vi "main.vi"() -> ()   [LabVIEW 2018]
uses:
  <vilib>/Analysis/NI_AALBase.lvlib
  <vilib>/Analysis/baseanly.llb/Real Inverse Matrix.vi
  <vilib>/robotics/Kinematics/Quaternion.ctl
  <vilib>/robotics/Kinematics/NI_Kinematics.lvlib
  <vilib>/imathl/engines/lvmath/Functions/Error Handling/Create Error.vi
  <vilib>/imath/engines/lvmath2/RunTimeEngine/IndexRead/NIMS V(S).vi
  <vilib>/imath/engines/lvmath2/RunTimeEngine/NodeEndStatement/NIMS_NodeEndStatement_Output.vi
  <vilib>/imath/engines/lvmath2/RunTimeEngine/ErrorHandling/NIMS_Finalize Error.vi
  <vilib>/imath/engines/lvmath2/RunTimeEngine/IndexRead/NIMS V(R2).vi
  <vilib>/imath/engines/lvmath2/RunTimeEngine/BuiltInFunctions/mean/NIMS_RS=mean(RV,I32).vi
  <vilib>/imath/engines/lvmath2/RunTimeEngine/IndexRead/NIMS M($,S).vi
  <vilib>/imath/engines/lvmath2/RunTimeEngine/RowToken/NIMS_RowToken_SorRV_CV.vi
panel:
  out "avg_er3":dbl
  out "avg_er2":dbl
  out "avg_er1":dbl
  out "eR (Yaw)":cluster{"E1_now":dbl[], "t_now":dbl[]}(graph)
  out "eR (Pitch)":cluster{"E1_now":dbl[], "t_now":dbl[]}(graph)
  out "eR (Roll)":cluster{"E1_now":dbl[], "t_now":dbl[]}(graph)
  out "Yaw":cluster{"E1_now":dbl[], "t_now":dbl[]}(graph)
  out "Pitch":cluster{"E1_now":dbl[], "t_now":dbl[]}(graph)
  out "Roll":cluster{"E1_now":dbl[], "t_now":dbl[]}(graph)
  in  "Simulation Time (sec)":dbl
  in  "Systems Configuration":T1
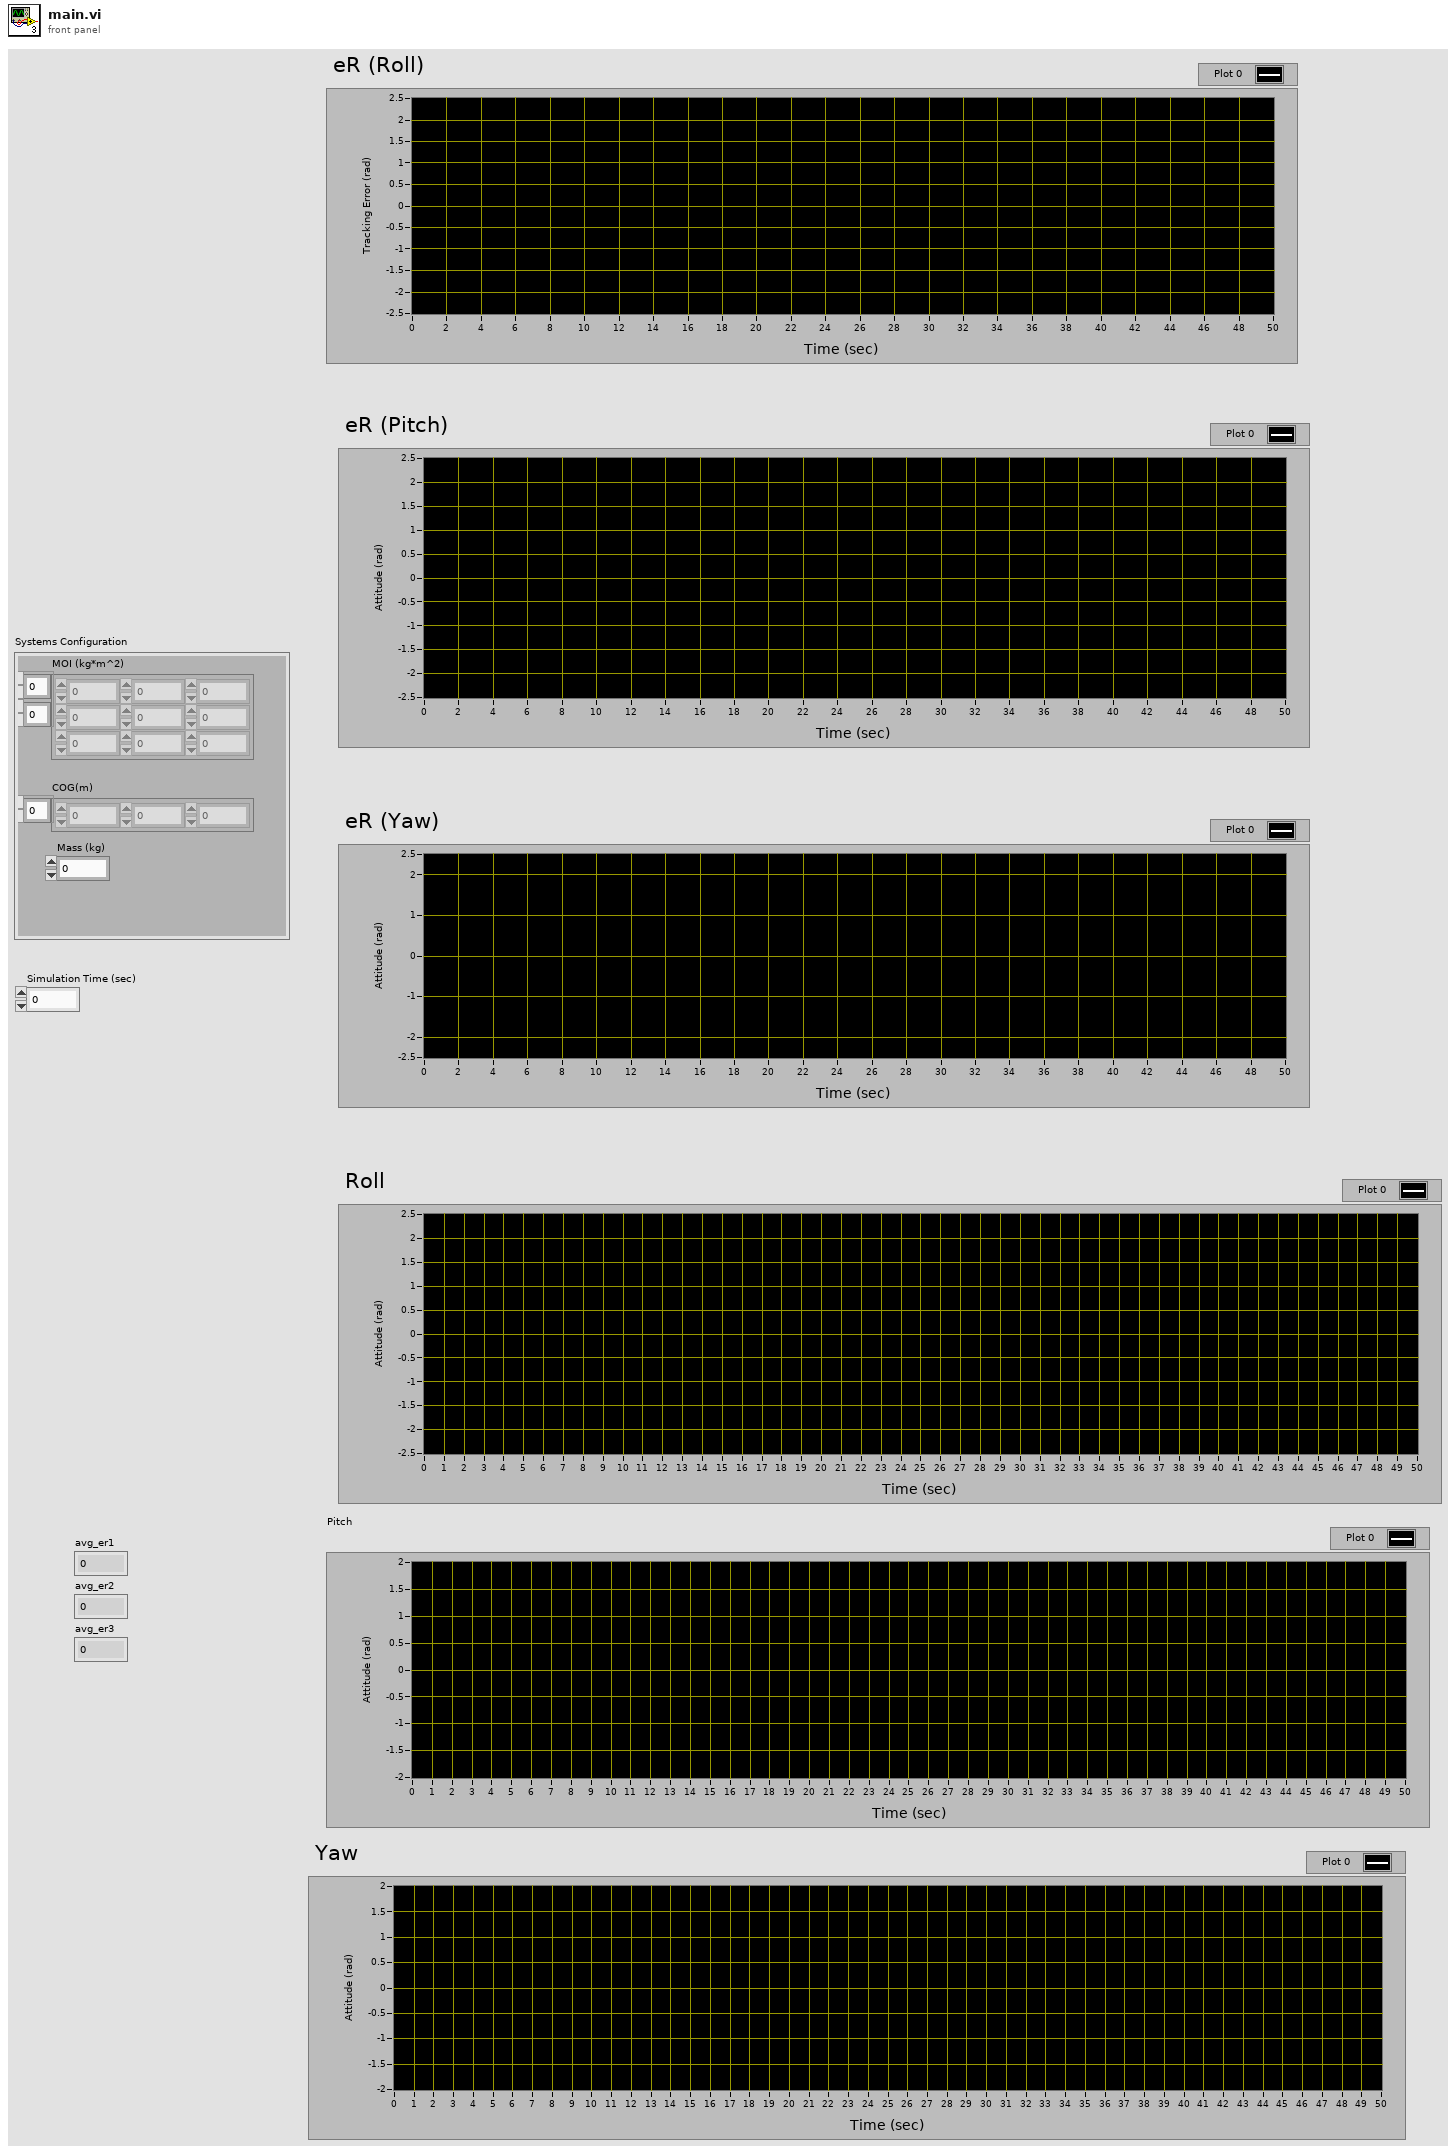
[diagram p1: front panel]
types:
  T1 = cluster{"MOI (kg*m^2)":dbl[][], "Mass (kg)":dbl, "COG(m)":dbl[]}
  T2 = typedef "NI_Matrix.lvlib/RealMatrix.ctl" = dbl[][]
  T3 = cluster{"MOI (kg*m^2)":dbl[][], "Inverse Matrix":T2, "Mass (kg)":dbl, "COG(m)":dbl[]}
  T4 = typedef "NI_Kinematics.lvlib/Quaternion.ctl" = dbl[]
  T5 = cluster{"E1_now":dbl[], "E2_now":dbl[], "E3_now":dbl[], "t_now":dbl[]}
  T6 = cluster{"Er1":dbl[], "Er2":dbl[], "Er3":dbl[], "t_now":dbl[]}
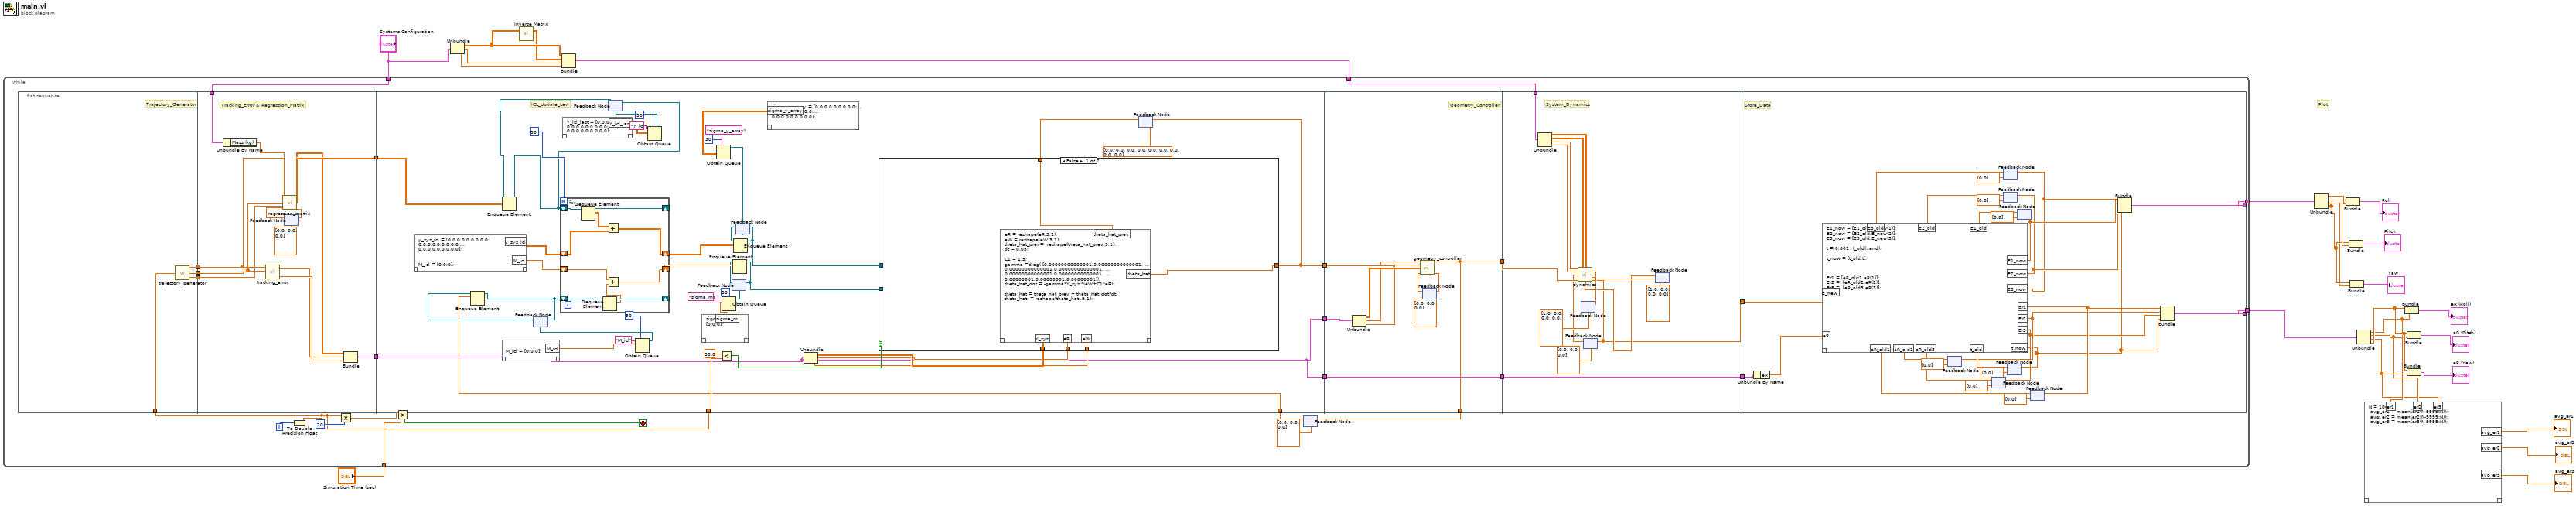
[diagram p0: block diagram]
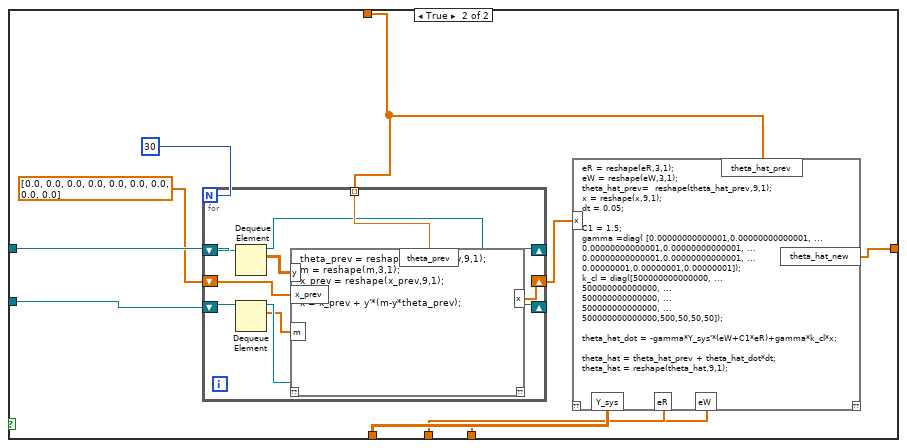
[diagram p2: hidden frame]
diagram:
  # "Plot"
  n1 = Unbundle("Systems Configuration") -> ("MOI (kg*m^2)"=w24:dbl[][], "Mass (kg)"=w22:dbl, "COG(m)"=w21:dbl[])
  n2 = call-poly <vilib>:"Inverse Matrix.vi"("Input Matrix"=w24) -> ("Inverse Matrix"=w23:T2)  [unwired: 1 in, 1 out]
  n3 = Bundle("MOI (kg*m^2)"=w24, "Inverse Matrix"=w23, "Mass (kg)"=w22, "COG(m)"=w21) -> (w20:T3)  [unwired: 1 in]
  n4 = while {
    tunnel: "Simulation Time (sec)" -> [w49]
    tunnel: "Systems Configuration" -> [w44]
    tunnel: w20 -> [w36]
    tunnel: [w31] -> w12
    tunnel: [w30] -> w1
    i -> [w47]
    stop <- w48 stop-if-true
    n5 = flat-sequence {
      tunnel: w41 -> [w55]
      tunnel: [w54] -> w46
      tunnel: [w53] -> w45
      tunnel: [w52] -> w43
      tunnel: w46 -> [w63]
      tunnel: w45 -> [w62]
      tunnel: w44 -> [w68]
      tunnel: w43 -> [w61]
      tunnel: [w60] -> w42
      tunnel: [w56] -> w40
      tunnel: w42 -> [w109]
      tunnel: w41 -> [w105]
      tunnel: w40 -> [w70]
      tunnel: [w70] -> w39
      tunnel: [w71] -> w38
      tunnel: [w70] -> w34
      tunnel: w28 -> [w69]
      tunnel: w39 -> [w153]
      tunnel: w38 -> [w148]
      tunnel: [w144] -> w37
      tunnel: w34 -> [w145]
      tunnel: [w145] -> w33
      tunnel: [w144] -> w29
      tunnel: w37 -> [w168]
      tunnel: w36 -> [w167]
      tunnel: [w155] -> w35
      tunnel: w33 -> [w154]
      tunnel: [w154] -> w32
      tunnel: w35 -> [w192]
      tunnel: w32 -> [w194]
      tunnel: [w170] -> w31
      tunnel: [w169] -> w30
      frame #0 {
        # "Trajectory_Generator"
        n6 = call "trajectory_generator.vi"("T"=w55) -> ("Ed"=w54:dbl[], "desired_angular_velocity"=w53:dbl[], "desired_angular_acceleration"=w52:dbl[])
      }
      frame #1 {
        # "Tracking_Error & Regression_Matrix"
        n7 = Unbundle By Name(w68) -> ("Mass (kg)"=w67:dbl)
        n8 = call "tracking_error.vi"("Ed(\"ZYX\")"=w63, "Wd"=w62) -> ("eR"=w58:dbl[], "eW"=w59:dbl[])  [unwired: 3 in]
        n9 = feedback #1(dbl[] [0.0, 0.0, 0.0] ("W_Prev")) -> (w65:dbl[])
        n10 = call "regression_matrix.vi"("m"=w67, "Ed"=w63, "Wd"=w62, "Wd_dot"=w61, "W_prev"=w65) -> ("Y_sys"=w57:dbl[][], "Y_icl_sys"=w60:dbl[][], "W_Prev"=w66:dbl[])  [unwired: 20 in]
        n11 = feedback-in #1(w66) -> ()
        n12 = Bundle("Y_sys"=w57, "eR"=w58, "eW"=w59) -> (w56:cluster{"Y_sys":dbl[][], "eR":dbl[], "eW":dbl[]})  [unwired: 1 in]
      }
      frame #2 {
        # "ICL_Update_Law"
        n13 = mathscript code="y_sys_icl = [0,0,0,0,0,0,0,0,0;...\n0,0,0,0,0,0,0,0,0;...\n0,0,0,0,0,0,0,0,0];\n\n\nM_icl = [0;0;0];"() -> ("y_sys_icl"=w107:dbl[][], "M_icl"=w106:dbl[])  [unwired: 1 in, 1 out]
        n14 = mathscript code="M_icl = [0;0;0];"() -> ("M_icl"=w95:dbl[])  [unwired: 1 in, 1 out]
        n15 = mathscript code="Y_icl_last = [0,0,0,0,0,0,0,0,0;...\n0,0,0,0,0,0,0,0,0;...\n0,0,0,0,0,0,0,0,0];"() -> ("Y_icl_last"=w100:dbl[][])  [unwired: 1 in, 1 out]
        n16 = Obtain Queue(max queue size (-1, unlimited)=30, name (unnamed)="M_icl", element data type=w95) -> (queue out=w94:refnum<queue>)  [unwired: 2 in, 2 out]
        n17 = feedback #2(w94) -> (w89:refnum<queue>)
        n18 = Enqueue Element(queue=w89, element=w69) -> (queue out=w90:refnum<queue>)  [unwired: 2 in, 2 out]
        n19 = feedback-in #2(w90) -> ()
        n20 = Obtain Queue(max queue size (-1, unlimited)=30, name (unnamed)="Y_icl", element data type=w100) -> (queue out=w99:refnum<queue>)  [unwired: 2 in, 2 out]
        n21 = feedback #3(w99) -> (w96:refnum<queue>)
        n22 = Enqueue Element(queue=w96, element=w109) -> (queue out=w91:refnum<queue>)  [unwired: 2 in, 2 out]
        n23 = for {
          N: 30 -> [_]
          shift-right: [w139] -> _
          shift-left: w91 -> [w143]
          shift-right: [w140] -> w102
          shift-left: w107 -> [w141]
          shift-right: [w137] -> w101
          shift-left: w106 -> [w138]
          shift-right: [w136] -> _
          shift-left: w90 -> [w135]
          n24 = Dequeue Element(queue=w143) -> (queue out=w139:refnum<queue>, element=w142:dbl[][])  [unwired: 2 in, 2 out]
          n25 = Dequeue Element(queue=w135) -> (queue out=w136:refnum<queue>, element=w134:dbl[])  [unwired: 2 in, 2 out]
          n26 = Add(x=w142, y=w141) -> (x+y=w140:dbl[][])
          n27 = Add(x=w138, y=w134) -> (x+y=w137:dbl[])
        }
        n28 = feedback-in #3(w91) -> ()
        n29 = mathscript code="sigma_m = [0;0;0];"() -> ("sigma_m"=w79:dbl[])  [unwired: 1 in, 1 out]
        n30 = Less?(x=30.0, y=w105) -> (x < y?=w103:bool)
        n31 = Obtain Queue(max queue size (-1, unlimited)=30, name (unnamed)="sigma_m", element data type=w79) -> (queue out=w80:refnum<queue>)  [unwired: 2 in, 2 out]
        n32 = feedback #4(w80) -> (w83:refnum<queue>)
        n33 = Enqueue Element(queue=w83, element=w101) -> (queue out=w72:refnum<queue>)  [unwired: 2 in, 2 out]
        n34 = feedback-in #4(w72) -> ()
        n35 = mathscript code="sigma_y_array = [0,0,0,0,0,0,0,0,0;...\n0,0,0,0,0,0,0,0,0;...\n0,0,0,0,0,0,0,0,0];"() -> ("sigma_y_array"=w88:dbl[][])  [unwired: 1 in, 1 out]
        n36 = Obtain Queue(max queue size (-1, unlimited)=30, name (unnamed)="sigma_y_array", element data type=w88) -> (queue out=w85:refnum<queue>)  [unwired: 2 in, 2 out]
        n37 = feedback #5(w85) -> (w84:refnum<queue>)
        n38 = Enqueue Element(queue=w84, element=w102) -> (queue out=w73:refnum<queue>)  [unwired: 2 in, 2 out]
        n39 = feedback-in #5(w73) -> ()
        n40 = Unbundle(w70) -> ("Y_sys"=w78:dbl[][], "eR"=w77:dbl[], "eW"=w76:dbl[])
        n41 = feedback #6(dbl[] [0.0, 0.0, 0.0, 0.0, 0.0, 0.0, 0.0, 0.0, 0.0] ("theta_hat")) -> (w74:dbl[])
        n42 = case shown="False" w103 {
          tunnel: w78 -> [w114 w124]
          tunnel: w77 -> [w113 w123]
          tunnel: w76 -> [w112 w122]
          tunnel: w74 -> [w111 w118]
          tunnel: w73 -> [_ w121]
          tunnel: w72 -> [_ w120]
          tunnel: [w110 w115] -> w71
          frame False {
            n43 = mathscript code="eR = reshape(eR,3,1);\neW = reshape(eW,3,1);\ntheta_hat_prev=  reshape(theta_hat_prev,9,1);\ndt = 0.05;\n\nC1 = 1.5;\ngamma =diag( [0.00000000000001,0.00000000000001, ...\n0.00000000000001,0.00000000000001, ...\n0.00000000000001,0.00000000000001, ...\n0.00000001,0.00000001,0.00000001]);\ntheta_hat_dot = -gamma*Y_sys'*(eW+C1*eR);\n\ntheta_hat = theta_hat_prev + theta_hat_dot*dt;\ntheta_hat  = reshape(theta_hat ,9,1);"("Y_sys"=w114, "eR"=w113, "eW"=w112, "theta_hat_prev"=w111) -> ("theta_hat"=w110:dbl[])  [unwired: 1 in, 1 out]
          }
          frame True {
            n44 = for {
              N: 30 -> [_]
              shift-right: [w130] -> _
              shift-left: w121 -> [w133]
              shift-right: [w129] -> _
              shift-left: w120 -> [w132]
              tunnel: w118 -> [w131] mode=indexing
              shift-right: [w125] -> w116
              shift-left: dbl[] [0.0, 0.0, 0.0, 0.0, 0.0, 0.0, 0.0, 0.0, 0.0] -> [w126]
              n45 = Dequeue Element(queue=w133) -> (queue out=w130:refnum<queue>, element=w128:dbl[][])  [unwired: 2 in, 2 out]
              n46 = Dequeue Element(queue=w132) -> (queue out=w129:refnum<queue>, element=w127:dbl[])  [unwired: 2 in, 2 out]
              n47 = mathscript code="theta_prev = reshape(theta_prev,9,1);\nm = reshape(m,3,1);\nx_prev = reshape(x_prev,9,1);\n\nx = x_prev + y'*(m-y*theta_prev);"("theta_prev"=w131, "y"=w128, "m"=w127, "x_prev"=w126) -> ("x"=w125:dbl[])  [unwired: 1 in, 1 out]
            }
            n48 = mathscript code="eR = reshape(eR,3,1);\neW = reshape(eW,3,1);\ntheta_hat_prev=  reshape(theta_hat_prev,9,1);\nx = reshape(x,9,1);\ndt = 0.05;\n\nC1 = 1.5;\ngamma =diag( [0.00000000000001,0.00000000000001, ...\n0.00000000000001,0.00000000000001, ...\n0.00000000000001,0.00000000000001, ...\n0.00000001,0.00000001,0.00000001]);\nk_cl = diag([500000000000000, ...\n500000000000000, ...\n500000000000000, ...\n500000000000000, ...\n500000000000000,500,50,50,50]);\n\ntheta_hat_dot = -gamma*Y_sys'*(eW+C1*eR)+gamma*k_cl*x;\n\ntheta_hat = theta_hat_prev + theta_hat_dot*dt;\ntheta_hat = reshape(theta_hat,9,1);"("Y_sys"=w124, "eR"=w123, "eW"=w122, "theta_hat_prev"=w118, "x"=w116) -> ("theta_hat_new"=w115:dbl[])  [unwired: 1 in, 1 out]
          }
        }
        n49 = feedback-in #6(w71) -> ()
      }
      frame #3 {
        # "Geometry_Controller"
        n50 = Unbundle(w153) -> ("Y_sys"=w152:dbl[][], "eR"=w146:dbl[], "eW"=w151:dbl[])
        n51 = feedback #7(dbl[] [0.0, 0.0, 0.0] ("Omega_now")) -> (w149:dbl[])
        n52 = call "geometry_controller.vi"("eR"=w146, "eW"=w151, "Y_sys"=w152, "theta_hat"=w148, "Omga_prev"=w149) -> ("M"=w144:dbl[], "Omega_now"=w150:dbl[])  [unwired: 9 in]
        n53 = feedback-in #7(w150) -> ()
      }
      frame #4 {
        # "System_Dynamics"
        n54 = Unbundle(w167) -> ("MOI (kg*m^2)"=w166:dbl[][], "Inverse Matrix"=w165:T2, "Mass (kg)"=w164:dbl, "COG(m)"=w163:dbl[])
        n55 = feedback #8(dbl[] [1.0, 0.0, 0.0, 0.0] ("W")) -> ()  [unwired: 1 in]
        n56 = feedback #9(dbl[] [0.0, 0.0, 0.0] ("E")) -> (w157:dbl[])
        n57 = feedback #10(T4 [1.0, 0.0, 0.0, 0.0] ("unit quaternion")) -> (w159:T4)
        n58 = call "dynamics.vi"("m"=w164, "J_inv"=w165, "J"=w166, "r"=w163, "E"=w157, "M"=w168, "q"=w159) -> ("W"=w162:dbl[], "unit quaternion"=w160:T4, "E"=w155:dbl[])  [unwired: 6 in]
        n59 = feedback-in #8(w162) -> ()
        n60 = feedback-in #9(w155) -> ()
        n61 = feedback-in #10(w160) -> ()
      }
      frame #5 {
        # "Store_Data"
        n62 = Unbundle By Name(w194) -> ("eR"=w193:dbl[])
        n63 = feedback #11(dbl[] [0.0] ("Er2")) -> (w187:dbl[])
        n64 = feedback #12(dbl[] [0.0] ("Er3")) -> (w189:dbl[])
        n65 = feedback #13(dbl[] [0.0] ("E3_now")) -> (w181:dbl[])
        n66 = feedback #14(dbl[] [0.0] ("E2_now")) -> (w182:dbl[])
        n67 = feedback #15(dbl[] [0.0] ("t_now")) -> (w191:dbl[])
        n68 = feedback #16(dbl[] [0.0] ("E1_now")) -> (w183:dbl[])
        n69 = feedback #17(dbl[] [0.0] ("Er1")) -> (w185:dbl[])
        n70 = mathscript code="E1_now = [E1_old,E_new(1)];\nE2_now = [E2_old,E_new(2)];\nE3_now = [E3_old,E_new(3)];\n\nt = 0.001+t_old(:,end);\n\nt_now = [t_old,t];\n\n\n\nEr1 = [eR_old1,eR(1)];\nEr2 =  [eR_old2,eR(2)];\nEr3 =  [eR_old3,eR(3)];"("E_new"=w192, "E1_old"=w183, "E2_old"=w182, "E3_old"=w181, "t_old"=w191, "eR"=w193, "eR_old1"=w185, "eR_old2"=w187, "eR_old3"=w189) -> ("E1_now"=w177:dbl[], "E2_now"=w176:dbl[], "E3_now"=w175:dbl[], "t_now"=w171:dbl[], "Er1"=w174:dbl[], "Er2"=w173:dbl[], "Er3"=w172:dbl[])  [unwired: 1 in, 1 out]
        n71 = feedback-in #11(w173) -> ()
        n72 = feedback-in #12(w172) -> ()
        n73 = feedback-in #13(w175) -> ()
        n74 = feedback-in #14(w176) -> ()
        n75 = feedback-in #15(w171) -> ()
        n76 = feedback-in #16(w177) -> ()
        n77 = feedback-in #17(w174) -> ()
        n78 = Bundle("E1_now"=w177, "E2_now"=w176, "E3_now"=w175, "t_now"=w171) -> (w170:T5)  [unwired: 1 in]
        n79 = Bundle("Er1"=w174, "Er2"=w173, "Er3"=w172, "t_now"=w171) -> (w169:T6)  [unwired: 1 in]
      }
    }
    n80 = To Double Precision Float(number=w47) -> (double precision float=w41:dbl)
    n81 = Multiply(x=w41, y=20) -> (x*y=w50:dbl)
    n82 = Greater?(x=w50, y=w49) -> (0:w48:bool)
    n83 = feedback-in #18(w29) -> ()
    n84 = feedback #18(dbl[] [0.0, 0.0, 0.0] ("M")) -> (w28:dbl[])
  }
  n85 = Unbundle(w12) -> ("E1_now"=w19:dbl[], "E2_now"=w18:dbl[], "E3_now"=w13:dbl[], "t_now"=w17:dbl[])
  n86 = Bundle("t_now"=w17, "E1_now"=w19) -> (→"Roll":cluster{"t_now":dbl[], "E1_now":dbl[]})  [unwired: 1 in]
  n87 = Bundle("t_now"=w17, "E2_now"=w18) -> (→"Pitch":cluster{"t_now":dbl[], "E2_now":dbl[]})  [unwired: 1 in]
  n88 = Bundle("t_now"=w17, "E3_now"=w13) -> (→"Yaw":cluster{"t_now":dbl[], "E3_now":dbl[]})  [unwired: 1 in]
  n89 = Unbundle(w1) -> ("Er1"=w7:dbl[], "Er2"=w6:dbl[], "Er3"=w5:dbl[], "t_now"=w8:dbl[])
  n90 = mathscript code="N = 10000;\n avg_er1 = mean(er1(N-9999:N));\n avg_er2 = mean(er2(N-9999:N));\n avg_er3 = mean(er3(N-9999:N));"("er1"=w7, "er2"=w6, "er3"=w5) -> ("avg_er1"=→"avg_er1":dbl, "avg_er2"=→"avg_er2":dbl, "avg_er3"=→"avg_er3":dbl)  [unwired: 1 in, 1 out]
  n91 = Bundle("t_now"=w8, "Er1"=w7) -> (→"eR (Roll)":cluster{"t_now":dbl[], "Er1":dbl[]})  [unwired: 1 in]
  n92 = Bundle("t_now"=w8, "Er2"=w6) -> (→"eR (Pitch)":cluster{"t_now":dbl[], "Er2":dbl[]})  [unwired: 1 in]
  n93 = Bundle("t_now"=w8, "Er3"=w5) -> (→"eR (Yaw)":cluster{"t_now":dbl[], "Er3":dbl[]})  [unwired: 1 in]
